vi "FRCts20_Backend_Initialize.vi"(8 "error in (no error)":errorcluster) -> (0 "error out":errorcluster, 3 "Engine_Refnums":T1)   [LabVIEW 2014, in "FRCts20_Backend_Engine.lvlib"]
doc: "The Initialize forms the data file path, as well \nas creates the Method and Return queue for\nuse during main processing operations."
uses:
  FRCts20_Backend_Engine.lvlib
  FRCts20_Backend_EngineRefnums.ctl
  INI_Accessor/FRCts20_Backend_INI Controller.lvclass
  Dependencies/AMC/_SubVIs/TypeDefs/Message Queue.ctl
  Dependencies/AMC/_SubVIs/TypeDefs/Message.ctl
  Dependencies/Keyed Array/KeyedArray.ctl
  <vilib>/addons/database/Connection.llb/Conn ObjectReference.ctl
  <vilib>/National Instruments/NI Amazon Web Services (AWS) Toolkit for LabVIEW/SNS/VI Source/AWS SNS Class/AWS_SNS.lvclass
  FRCts20_Backend_Dyn_FGV_Command.ctl
  <vilib>/addons/database/Connection.llb/DB Tools Open Connec (String).vi
  Dependencies/AMC/AMC.lvlib
  Dependencies/Keyed Array/Tools_KeyedArray.lvlib
  <vilib>/addons/database/NI_Database_API.lvlib
panel:
  # "Creates the Method and Return queue for\nuse during main processing operations.\nOpens connection to db"
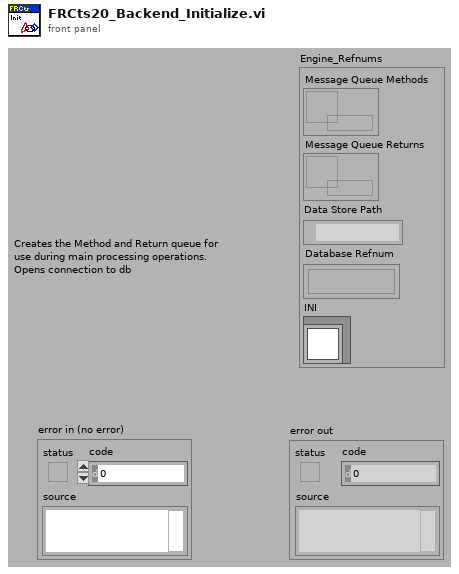
[diagram p1: front panel]
types:
  T1 = typedef "FRCts20_Backend_Engine.lvlib/FRCts20_Backend_EngineRefnums.ctl" = cluster{"Message Queue Methods":T2, "Message Queue Returns":T2, "Data Store Path":path, "Database Refnum":T3, "INI":refnum<class "FRCts20_Backend_INI Controller.lvclass">}
  T2 = typedef "AMC.lvlib/Message Queue.ctl" = refnum<queue>
  T3 = typedef "NI_Database_API.lvlib/Conn ObjectReference.ctl" = refnum<k1>
  T4 = typedef "FRCts20_Backend_Engine.lvlib/FRCts20_Backend_Dyn_FGV_Command.ctl" = enum16{"Load", "Locate", "Unload"}
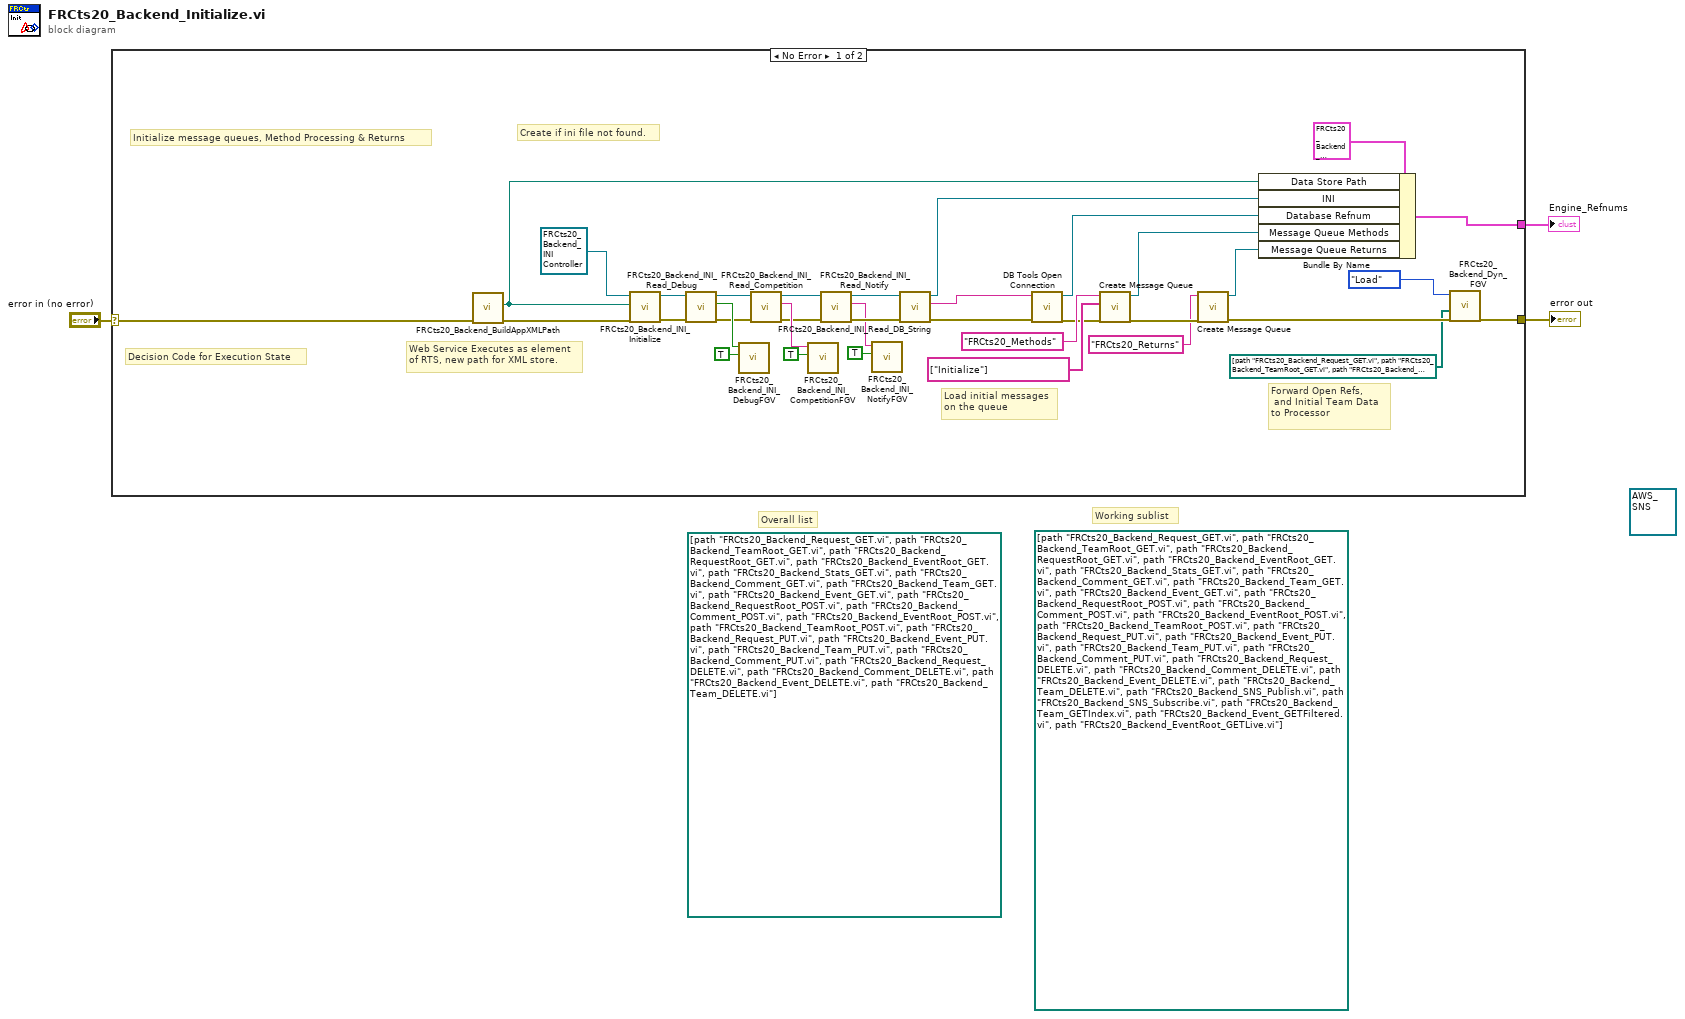
[diagram p0: block diagram]
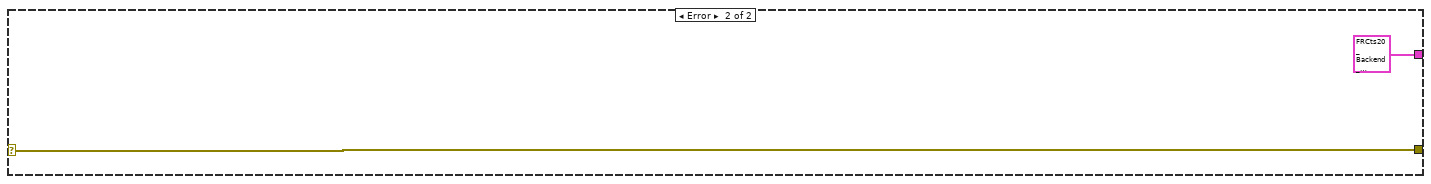
[diagram p2: hidden frame]
diagram:
  (unwired) refnum<class "AWS_SNS.lvclass"> refnum ("AWS_SNS.lvlib:AWS_SNS.lvclass")
  (unwired) path[] [path "FRCts20_Backend_Request_GET.vi", path "FRCts20_Backend_TeamRoot_GET.vi", path "FRCts20_Backend_RequestRoot_GET.vi", path "FRCts20_Backend_EventRoot_GET.vi", path "FRCts20_Backend_Stats_GET.vi", path "FRCts20_Backend_Comment_GET.vi", path "FRCts20_Backend_Team_GET.vi", path "FRCts20_Backend_Event_GET.vi", path "FRCts20_Backend_RequestRoot_POST.vi", path "FRCts20_Backend_Comment_POST.vi", path "FRCts20_Backend_EventRoot_POST.vi", path "FRCts20_Backend_TeamRoot_POST.vi", path "FRCts20_Backend_Request_PUT.vi", path "FRCts20_Backend_Event_PUT.vi", path "FRCts20_Backend_Team_PUT.vi", path "FRCts20_Backend_Comment_PUT.vi", path "FRCts20_Backend_Request_DELETE.vi", path "FRCts20_Backend_Comment_DELETE.vi", path "FRCts20_Backend_Event_DELETE.vi", path "FRCts20_Backend_Team_DELETE.vi"] ("VI Names")
  (unwired) path[] [path "FRCts20_Backend_Request_GET.vi", path "FRCts20_Backend_TeamRoot_GET.vi", path "FRCts20_Backend_RequestRoot_GET.vi", path "FRCts20_Backend_EventRoot_GET.vi", path "FRCts20_Backend_Stats_GET.vi", path "FRCts20_Backend_Comment_GET.vi", path "FRCts20_Backend_Team_GET.vi", path "FRCts20_Backend_Event_GET.vi", path "FRCts20_Backend_RequestRoot_POST.vi", path "FRCts20_Backend_Comment_POST.vi", path "FRCts20_Backend_EventRoot_POST.vi", path "FRCts20_Backend_TeamRoot_POST.vi", path "FRCts20_Backend_Request_PUT.vi", path "FRCts20_Backend_Event_PUT.vi", path "FRCts20_Backend_Team_PUT.vi", path "FRCts20_Backend_Comment_PUT.vi", path "FRCts20_Backend_Request_DELETE.vi", path "FRCts20_Backend_Comment_DELETE.vi", path "FRCts20_Backend_Event_DELETE.vi", path "FRCts20_Backend_Team_DELETE.vi", path "FRCts20_Backend_SNS_Publish.vi", path "FRCts20_Backend_SNS_Subscribe.vi", path "FRCts20_Backend_Team_GETIndex.vi", path "FRCts20_Backend_Event_GETFiltered.vi", path "FRCts20_Backend_EventRoot_GETLive.vi"] ("VI Names")
  # "Working sublist"
  # "Overall list"
  n1 = case shown="No Error" "error in (no error)" {
    selector: "error in (no error)" -> [w21 w40]
    tunnel: [w28 w40] -> w2
    tunnel: [w31 T1 {"Message Queue Methods"=refnum, "Message Queue Returns"=refnum, "Data Store Path"=path "", "Database Refnum"=refnum, "INI"=refnum} ("Engine_Refnums Const")] -> w1
    frame No Error {
      # "Web Service Executes as element\nof RTS, new path for XML store."
      # "Forward Open Refs,\n and Initial Team Data \nto Processor"
      # "Create if ini file not found."
      # "Load initial messages\non the queue"
      # "Decision Code for Execution State"
      # "Initialize message queues, Method Processing & Returns"
      n2 = call "FRCts20_Backend_BuildAppXMLPath.vi"("error in (no error)"=w21) -> ("error out"=w20:errorcluster, "Path Out"=w23:path)  [unwired: 9 in]
      n3 = call "FRCts20_Backend_INI_Initialize.vi"("error in (no error)"=w20, "Config Path"=w23, "INI Controller in"=refnum<class "FRCts20_Backend_INI Controller.lvclass"> refnum ("FRCts20_Backend_Engine.lvlib:FRCts20_Backend_INI Controller.lvclass")) -> ("error out"=w17:errorcluster, "INI Controller out"=w18:refnum<class "FRCts20_Backend_INI Controller.lvclass">)  [unwired: 7 in]
      n4 = call "FRCts20_Backend_INI_Read_Debug.vi"("error in (no error)"=w17, "INI Controller in"=w18) -> ("error out"=w14:errorcluster, "debug?"=w16:bool, "INI Controller out"=w13:refnum<class "FRCts20_Backend_INI Controller.lvclass">)  [unwired: 7 in]
      n5 = call "FRCts20_Backend_INI_DebugFGV.vi"("Set?"=TRUE, "Value in"=w16) -> ()  [unwired: 9 in, 1 out]
      n6 = call "FRCts20_Backend_INI_Read_Competition.vi"("error in (no error)"=w14, "INI Controller in"=w13) -> ("error out"=w10:errorcluster, "Competition Name"=w12:string, "INI Controller out"=w9:refnum<class "FRCts20_Backend_INI Controller.lvclass">)  [unwired: 7 in]
      n7 = call "FRCts20_Backend_INI_CompetitionFGV.vi"("Set?"=TRUE, "Value in"=w12) -> ()  [unwired: 9 in, 1 out]
      n8 = call "FRCts20_Backend_INI_Read_Notify.vi"("error in (no error)"=w10, "INI Controller in"=w9) -> ("error out"=w7:errorcluster, "Notify List"=w6:string, "INI Controller out"=w8:refnum<class "FRCts20_Backend_INI Controller.lvclass">)  [unwired: 7 in]
      n9 = call "FRCts20_Backend_INI_NotifyFGV.vi"("Set?"=TRUE, "Value in"=w6) -> ()  [unwired: 9 in, 1 out]
      n10 = call "FRCts20_Backend_INI_Read_DB_String.vi"("error in (no error)"=w7, "INI Controller in"=w8) -> ("error out"=w25:errorcluster, "Connection String"=w24:string, "INI Controller out"=w22:refnum<class "FRCts20_Backend_INI Controller.lvclass">)  [unwired: 7 in]
      n11 = call-poly <vilib>:"DB Tools Open Connection.vi"("error in (no error)"=w25, "connection information"=w24) -> ("error out"=w30:errorcluster, "connection reference"=w29:T3)  [unwired: 6 in]
      n12 = call "Create Message Queue.vi"("error in (no error)"=w30, "Initial Message Names"=string[] ["Initialize"], "Message Queue Name"="FRCts20_Methods" ("string")) -> ("error out"=w37:errorcluster, "Message Queue out"=w33:T2)  [unwired: 1 in, 6 out]
      n13 = call "Create Message Queue.vi"("error in (no error)"=w37, "Message Queue Name"="FRCts20_Returns" ("string")) -> ("error out"=w27:errorcluster, "Message Queue out"=w32:T2)  [unwired: 2 in, 6 out]
      n14 = Bundle By Name(cluster=T1 {"Message Queue Methods"=refnum, "Message Queue Returns"=refnum, "Data Store Path"=path "", "Database Refnum"=refnum, "INI"=refnum} ("Engine_Refnums Const"), "Data Store Path"=w23, "INI"=w22, "Database Refnum"=w29, "Message Queue Methods"=w33, "Message Queue Returns"=w32) -> (w31:T1)
      n15 = call "FRCts20_Backend_Dyn_FGV.vi"("error in"=w27, "VI List"=path[] [path "FRCts20_Backend_Request_GET.vi", path "FRCts20_Backend_TeamRoot_GET.vi", path "FRCts20_Backend_RequestRoot_GET.vi", path "FRCts20_Backend_EventRoot_GET.vi", path "FRCts20_Backend_Stats_GET.vi", path "FRCts20_Backend_Comment_GET.vi", path "FRCts20_Backend_Team_GET.vi", path "FRCts20_Backend_Event_GET.vi", path "FRCts20_Backend_RequestRoot_POST.vi", path "FRCts20_Backend_Comment_POST.vi", path "FRCts20_Backend_EventRoot_POST.vi", path "FRCts20_Backend_TeamRoot_POST.vi", path "FRCts20_Backend_Request_PUT.vi", path "FRCts20_Backend_Event_PUT.vi", path "FRCts20_Backend_Team_PUT.vi", path "FRCts20_Backend_Comment_PUT.vi", path "FRCts20_Backend_Request_DELETE.vi", path "FRCts20_Backend_Comment_DELETE.vi", path "FRCts20_Backend_Event_DELETE.vi", path "FRCts20_Backend_Team_DELETE.vi"] ("VI Names"), "Command"=FRCts20_Backend_Dyn_FGV_Command."Load") -> ("error out"=w28:errorcluster)  [unwired: 6 in, 2 out]
    }
    frame Error {
    }
  }
  "error out" <- w2
  "Engine_Refnums" <- w1
